vi "Refnum_control_global_BM.vi"() -> ()   [LabVIEW 2021]
panel:
  out "Refnum_control":bool
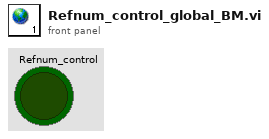
[diagram p1: front panel]
diagram:
